vi "inner_vi.vi"(11 "Bool Refnum":refnum<vi>) -> ()   [LabVIEW 2011]
panel:
  out "Value":bool
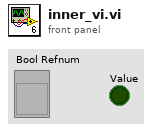
[diagram p1: front panel]
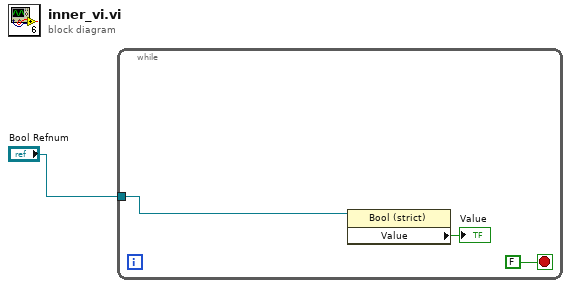
[diagram p0: block diagram]
diagram:
  n1 = while {
    tunnel: "Bool Refnum" -> [w3]
    stop <- FALSE stop-if-true
    n2 = property class="Bool (strict)"(reference=w3) -> ("Value"=→"Value":bool)  [unwired: 1 in, 2 out]
  }
